vi "Read_Ini_File.vi"(8 "Error In":errorcluster, 9 "Emotion":T1(ring), 11 "Type data":enum16{"I32", "Boolean"}(ring)) -> (0 "Error Out":errorcluster, 1 "Numeric_Array":i32[](array[numeric]), 2 "Boolean_Array":bool[](array[boolean]))   [LabVIEW 2017]
doc: "This Vi read from an .ini file.\n\nIt returns the configuration information.\n\nData type entries :\n-I32\n-Boolean"
uses:
  <vilib>/Utility/config.llb/Read Key (I32).vi
  <vilib>/Utility/config.llb/Read Key (Boolean).vi
  <vilib>/Utility/config.llb/NI_LVConfig.lvlib
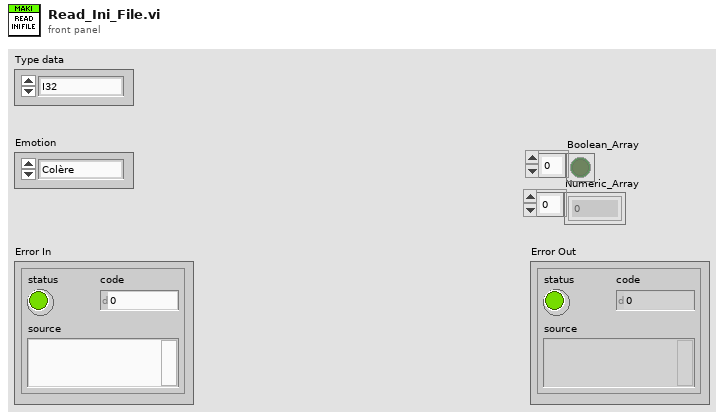
[diagram p1: front panel]
types:
  T1 = enum16{"Colère", "Suspicieux", "Fatigué", "Surpris", "Blasé", "Drôle", "Content", "Triste", "Clind'oeil"}
  T2 = typedef "NI_LVConfig.lvlib/Config Data RefNum.ctl" = refnum<k1>
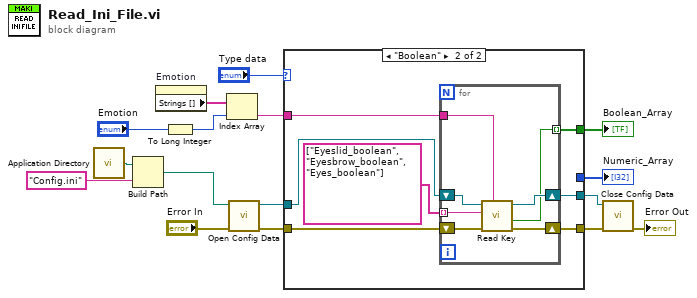
[diagram p0: block diagram]
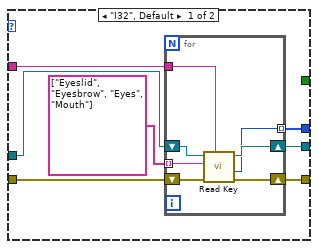
[diagram p2: hidden frame]
diagram:
  n1 = call <vilib>:"Application Directory.vi"() -> ("Application Directory"=w3:path)
  n2 = Build Path(base path=w3, name or relative path="Config.ini") -> (appended path=w1:path)
  n3 = property on="Emotion" class="Enum (strict)"() -> ("Strings []"=w6:string[])  [unwired: 2 in, 2 out]
  n4 = To Long Integer(number="Emotion") -> (32bit integer=w4:i32)
  n5 = Index Array(array=w6, index=w4) -> (element=w5:string)
  n6 = call <vilib>:"Open Config Data.vi"("error in (no error)"="Error In", "configuration file path"=w1) -> ("error out"=w11:errorcluster, "refnum"=w14:T2)  [unwired: 7 in, 1 out]
  n7 = case shown="\"Boolean\"" "Type data" {
    tunnel: w14 -> [w23 w37]
    tunnel: [w22 w36] -> w13
    tunnel: [w21 w35] -> w12
    tunnel: w11 -> [w20 w34]
    tunnel: [w19 _] -> w9
    tunnel: [_ w32] -> w8
    tunnel: w5 -> [w17 w31]
    frame "I32", Default {
      n8 = for {
        tunnel: [w26] -> w19 mode=indexing
        shift-right: [w29] -> w22
        shift-left: w23 -> [w30]
        shift-right: [w28] -> w21
        shift-left: w20 -> [w27]
        tunnel: string[] ["Eyeslid", "Eyesbrow", "Eyes", "Mouth"] -> [w25] mode=indexing
        tunnel: w17 -> [w24]
        n9 = call-poly <vilib>:"Read Key.vi"("section"=w24, "error in (no error)"=w27, "key"=w25, "refnum"=w30) -> ("error out"=w28:errorcluster, "value"=w26:i32, "refnum out"=w29:T2)  [unwired: 4 in, 1 out]
      }
    }
    frame "Boolean" {
      n10 = for {
        tunnel: [w40] -> w32 mode=indexing
        shift-right: [w43] -> w36
        shift-left: w37 -> [w44]
        shift-right: [w42] -> w35
        shift-left: w34 -> [w41]
        tunnel: string[] ["Eyeslid_boolean", "Eyesbrow_boolean", "Eyes_boolean"] -> [w39] mode=indexing
        tunnel: w31 -> [w38]
        n11 = call-poly <vilib>:"Read Key.vi"("section"=w38, "error in (no error)"=w41, "key"=w39, "refnum"=w44) -> ("error out"=w42:errorcluster, "value"=w40:bool, "refnum out"=w43:T2)  [unwired: 4 in, 1 out]
      }
    }
  }
  "Numeric_Array" <- w9
  "Boolean_Array" <- w8
  n12 = call <vilib>:"Close Config Data.vi"("error in (no error)"=w12, "refnum"=w13) -> ("error out"=→"Error Out":errorcluster)  [unwired: 8 in, 1 out]
